vi "ROI entry-Init UI elements.vi"(8 "error in (no error)":errorcluster) -> (0 "error out":errorcluster)   [LabVIEW 2013]
uses:
  Typedefs/ROI ID Enum.ctl
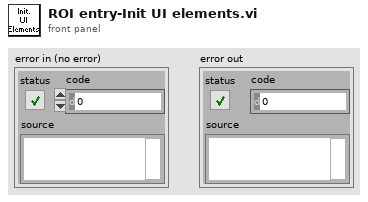
[diagram p1: front panel]
types:
  T1 = enum8{"Enabled", "Disabled", "Disabled and Grayed Out"}
  T2 = typedef "ROI ID Enum.ctl" = enum16{"Point", "MiniScan", "Comp. MiniScan", "Rectangle", "Comp. volume", "Arb. plane point"}
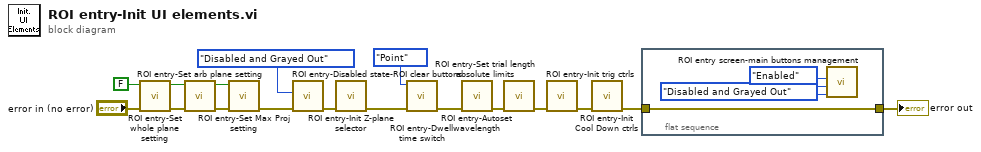
[diagram p0: block diagram]
diagram:
  w10 = FALSE ("Whole plane")
  n1 = call "ROI entry-Set whole plane setting.vi"("error in (no error)"="error in (no error)", "\"Whole plane\" button's value"=w10) -> ("error out"=w11:errorcluster)  [unwired: 9 in]
  n2 = call "ROI entry-Set arb plane setting.vi"("error in (no error)"=w11, "\"Arb plane entry\" button's value"=w10) -> ("error out"=w9:errorcluster)  [unwired: 9 in]
  n3 = call "ROI entry-Set Max Proj setting.vi"("error in (no error)"=w9, "Max Z-projection button value"=w10) -> ("error out"=w12:errorcluster)  [unwired: 9 in]
  n4 = call "ROI entry-Disabled state-ROI clear buttons.vi"("error in (no error)"=w12, "State"=T1."Disabled and Grayed Out" ("Disabled")) -> ("error out"=w8:errorcluster)  [unwired: 9 in]
  n5 = call "ROI entry-Init Z-plane selector.vi"("error in (no error)"=w8) -> ("error out"=w4:errorcluster)  [unwired: 10 in]
  n6 = call "ROI entry-Dwell time switch.vi"("error in (no error)"=w4, "ROI Enum"=ROI_ID_Enum."Point") -> ("error out"=w13:errorcluster)  [unwired: 9 in]
  n7 = call "ROI entry-Autoset wavelength.vi"("error in (no error)"=w13) -> ("error out"=w5:errorcluster)  [unwired: 10 in]
  n8 = call "ROI entry-Set trial length absolute limits.vi"("error in (no error)"=w5) -> ("error out"=w3:errorcluster)  [unwired: 10 in]
  n9 = call "ROI entry-Init trig ctrls.vi"("error in (no error)"=w3) -> ("error out"=w2:errorcluster)  [unwired: 10 in]
  n10 = call "ROI entry-Init Cool Down ctrls.vi"("error in (no error)"=w2) -> ("error out"=w1:errorcluster)  [unwired: 10 in]
  n11 = flat-sequence {
    tunnel: w1 -> [w16]
    tunnel: [w16] -> w15
    frame #0 {
      w18 = T1."Disabled and Grayed Out" ("Disabled")
      n12 = call "ROI entry screen-main buttons management.vi"("Imaging button disabled?"=w18, "Acquisition button disabled?"=w18, "Done button disabled?"=T1."Enabled" ("Disabled")) -> ()  [unwired: 9 in]
    }
  }
  "error out" <- w15
